vi "Configure DUT Mode.vi"(8 "error in (no error)":errorcluster, 9 "DUT Mode (0)":i16 min=0 max=1 step=1, 11 "VISA resource name":refnum<visa-resource-name>) -> (0 "error out":errorcluster, 3 "VISA resource name out":refnum<visa-resource-name>)   [LabVIEW 2012, in "Temptronic TP04300.lvlib"]
doc: "This VI configures DUT mode of TP04300 instrument.\n<b>DUT Mode</b> - used to configure the DUT Mode as follows:\n 0 - Air Modes\n 1 - DUT Mode\n\nDefault Value: 0 \nValid Range: 0 - 1"
uses:
  <instrlib>/Temptronic TP04300/Temptronic TP04300.lvlib
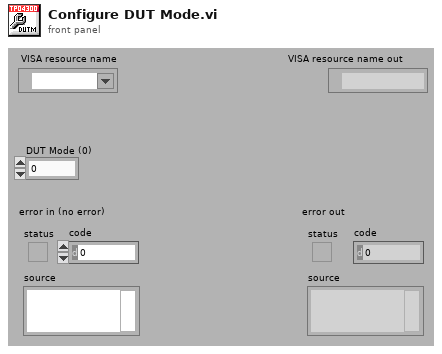
[diagram p1: front panel]
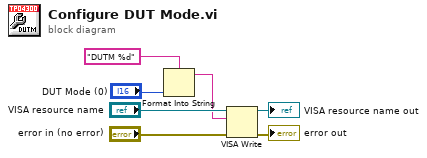
[diagram p0: block diagram]
diagram:
  n1 = Format Into String(format string="DUTM %d" ("multi-line string"), "DUT Mode (0)") -> (resulting string=w3:string)  [unwired: 2 in, 1 out]
  n2 = VISA Write(VISA resource name="VISA resource name", write buffer=w3, error in (no error)="error in (no error)") -> (VISA resource name out=→"VISA resource name out":refnum<visa-resource-name>, error out=→"error out":errorcluster)  [unwired: 1 out]
